vi "Arm_RLE_To_XYZ.vi"(9 "Extend":dbl, 10 "Lift":dbl, 11 "Rotate":dbl) -> (1 "z":dbl, 2 "y":dbl, 3 "x":dbl)   [LabVIEW 2020]
uses:
  <vilib>/Rock Robotics/WPI/ThirdParty/JAS_Junk/TrajLib/Trajectory_Library.lvlib
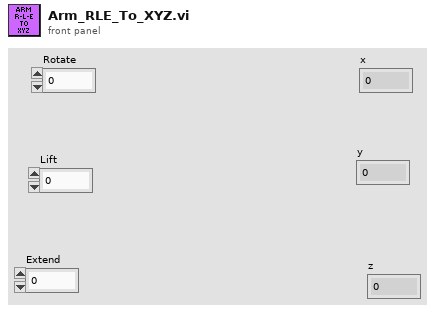
[diagram p1: front panel]
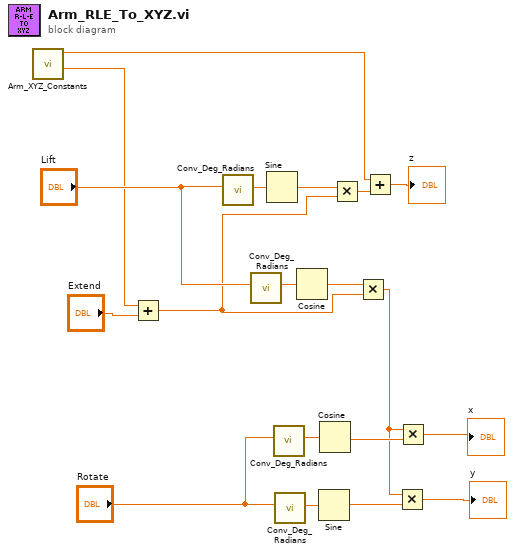
[diagram p0: block diagram]
diagram:
  n1 = call "Arm_XYZ_Constants.vi"() -> ("Unextended Length (in)"=w1:dbl, "Pivot Height (in)"=w2:dbl)  [unwired: 10 in]
  n2 = Add(x=w1, y="Extend") -> (x+y=w13:dbl)
  n3 = call <vilib>:"Conv_Deg_Radians.vi"("Degress"="Lift") -> ("Radians"=w19:dbl)  [unwired: 10 in]
  n4 = call <vilib>:"Conv_Deg_Radians.vi"("Degress"="Lift") -> ("Radians"=w16:dbl)  [unwired: 10 in]
  n5 = Sine(x=w19) -> (sin(x)=w17:dbl)
  n6 = call <vilib>:"Conv_Deg_Radians.vi"("Degress"="Rotate") -> ("Radians"=w11:dbl)  [unwired: 10 in]
  n7 = call <vilib>:"Conv_Deg_Radians.vi"("Degress"="Rotate") -> ("Radians"=w12:dbl)  [unwired: 10 in]
  n8 = Cosine(x=w16) -> (cos(x)=w14:dbl)
  n9 = Sine(x=w12) -> (sin(x)=w8:dbl)
  n10 = Cosine(x=w11) -> (cos(x)=w7:dbl)
  n11 = Multiply(x=w17, y=w13) -> (x*y=w4:dbl)
  n12 = Multiply(x=w14, y=w13) -> (x*y=w5:dbl)
  n13 = Add(x=w2, y=w4) -> (x+y=→"z":dbl)
  n14 = Multiply(x=w5, y=w8) -> (x*y=→"y":dbl)
  n15 = Multiply(x=w5, y=w7) -> (x*y=→"x":dbl)
